vi "Ramp PSU to Target.vi"(8 "error in (no error)":errorcluster, 9 "Target Rate (T/min)":dbl, 10 "Target Field (T)":dbl, 11 "Instrument.Oxford1820 in":refnum<class "Instrument.Oxford1820.lvclass">) -> (0 "error out":errorcluster, 3 "Instrument.Oxford1820 out":refnum<class "Instrument.Oxford1820.lvclass">)   [LabVIEW 2016, in "Instrument.Oxford1820.lvclass"]
uses:
  Instrument.Oxford1820.lvclass
  <instrlib>/Mercury iXX/Public/Libraries/Magnet/Controls/PSU Actions.ctl
  <instrlib>/Mercury iXX/Public/Libraries/Magnet.lvlib
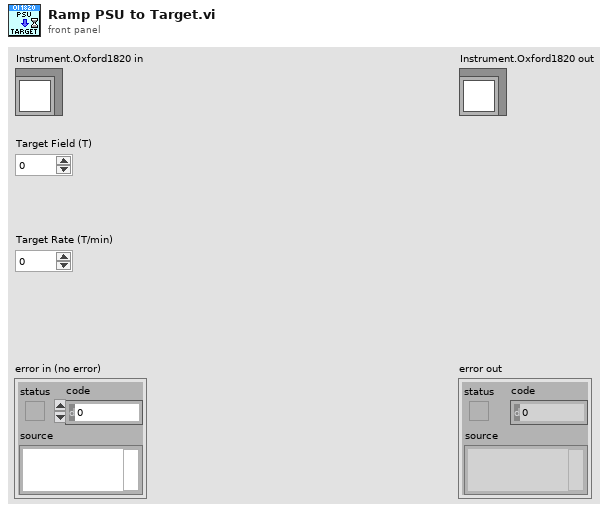
[diagram p1: front panel]
types:
  T1 = typedef "Mercury iXX.lvlib/Magnet.lvlib/PSU Actions.ctl" = string
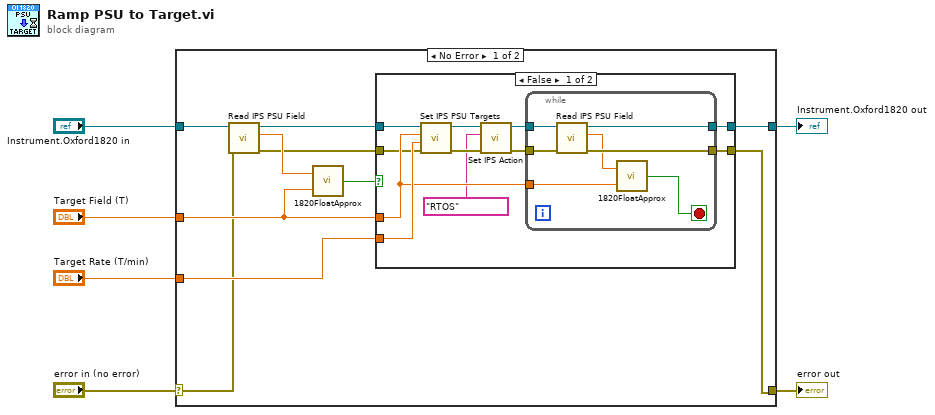
[diagram p0: block diagram]
diagram:
  n1 = case shown="No Error" "error in (no error)" {
    selector: "error in (no error)" -> [w8 w38]
    tunnel: [w15 w38] -> w5
    tunnel: [w16 w37] -> w3
    tunnel: "Instrument.Oxford1820 in" -> [w10 w37]
    tunnel: "Target Field (T)" -> [w13 _]
    tunnel: "Target Rate (T/min)" -> [w12 _]
    frame No Error {
      n2 = call "Read IPS PSU Field.vi"("error in (no error)"=w8, "Instrument.Oxford1820 in"=w10) -> ("error out"=w7:errorcluster, "Power Supply Field (T)"=w11:dbl, "Instrument.Oxford1820 out"=w9:refnum<class "Instrument.Oxford1820.lvclass">)  [unwired: 7 in]
      n3 = call "1820FloatApprox.vi"("y"=w13, "x"=w11) -> ("x ~ y?"=w14:bool)
      n4 = case shown="False" w14 {
        tunnel: [w27 w36] -> w16
        tunnel: [w26 w35] -> w15
        tunnel: w9 -> [w23 w36]
        tunnel: w7 -> [w22 w35]
        tunnel: w13 -> [w24 _]
        tunnel: w12 -> [w25 _]
        frame False {
          n5 = call "Set IPS PSU Targets.vi"("error in (no error)"=w22, "Target Field Rate (T/min)"=w25, "Target Field (T)"=w24, "Instrument.Oxford1820 in"=w23) -> ("error out"=w21:errorcluster, "Instrument.Oxford1820 out"=w20:refnum<class "Instrument.Oxford1820.lvclass">)  [unwired: 5 in, 1 out]
          n6 = call "Set IPS Action.vi"("error in (no error)"=w21, "PSU Act Stat"=T1 "RTOS", "Instrument.Oxford1820 in"=w20) -> ("error out"=w19:errorcluster, "Instrument.Oxford1820 out"=w18:refnum<class "Instrument.Oxford1820.lvclass">)  [unwired: 6 in, 1 out]
          n7 = while {
            tunnel: w19 -> [w32]
            tunnel: w18 -> [w31]
            tunnel: w24 -> [w34]
            tunnel: [w29] -> w27
            tunnel: [w30] -> w26
            stop <- w33 stop-if-true
            n8 = call "Read IPS PSU Field.vi"("error in (no error)"=w32, "Instrument.Oxford1820 in"=w31) -> ("error out"=w30:errorcluster, "Power Supply Field (T)"=w28:dbl, "Instrument.Oxford1820 out"=w29:refnum<class "Instrument.Oxford1820.lvclass">)  [unwired: 7 in]
            n9 = call "1820FloatApprox.vi"("y"=w34, "x"=w28) -> ("x ~ y?"=w33:bool)
          }
        }
        frame True {
          # "If PSU Field == Target, do nothing"
        }
      }
    }
    frame Error {
    }
  }
  "error out" <- w5
  "Instrument.Oxford1820 out" <- w3
